vi "Read Sweep Configuration Example.vi"   [LabVIEW 2019, in "SMO.SweepControl.lvclass"]
uses:
  SMO.SweepControl.lvclass
  Typedefs/Enum - Experiments.ctl
  Typedefs/Continuous B Sweep JSON--Cluster.ctl
  Typedefs/Enum - Priority.ctl
  Typedefs/Enum - Action.ctl
  Typedefs/Cluster - ScanControl.ctl
  Typedefs/ScanControl.ctl
  Typedefs/Cluster - ScanParamters.ctl
  Typedefs/ScanParamters.ctl
  Typedefs/Sweep Control JSON--Cluster.ctl
  SMO.Transport/Typedefs/Lockin_Sweep JSON--Cluster.ctl
  SMO.Transport/SMO.Transport.lvclass
  <userlib>/LevyLab/Krohn Hite 7008/typedefs/Input Configuration-Enum.ctl
  <userlib>/LevyLab/Krohn Hite 7008/Instrument.KH7008.lvclass
  <userlib>/LevyLab/Krohn Hite 7008/typedefs/Shunt-Enum.ctl
  <userlib>/LevyLab/Krohn Hite 7008/typedefs/Gain-Enum.ctl
  <userlib>/LevyLab/Krohn Hite 7008/typedefs/Channel-Enum.ctl
  <userlib>/LevyLab/Krohn Hite 7008/typedefs/Coupling-Enum.ctl
  <userlib>/LevyLab/Krohn Hite 7008/typedefs/Filter-Enum.ctl
  <userlib>/LevyLab/Krohn Hite 7008/typedefs/SetAll-Cluster.ctl
  <userlib>/LevyLab/Krohn Hite 7008/typedefs/SetAll-Array.ctl
  <userlib>/LevyLab/Lockin-Multichannel/Instrument.DAQ/Typedefs/REF.Channel--Cluster.ctl
  <userlib>/LevyLab/Lockin-Multichannel/Instrument.DAQ/Instrument.DAQ.lvclass
  <userlib>/LevyLab/Lockin-Multichannel/Instrument.DAQ/Typedefs/REF.Channel--Cluster--Array.ctl
  <userlib>/LevyLab/Lockin-Multichannel/Instrument.DAQ/Typedefs/AO.Channel.Function--Enum.ctl
  <userlib>/LevyLab/Lockin-Multichannel/Instrument.DAQ/Typedefs/AO.Channel--Cluster.ctl
  <userlib>/LevyLab/Lockin-Multichannel/Instrument.DAQ/Typedefs/AO.Channel--Cluster--Array.ctl
  Control Experiment/Typedefs/Wiring Description--v2--cluster.ctl
  Control Experiment/Control Experiment.lvclass
  Control Experiment/Typedefs/Instrument Types--combo.ctl
  Control Experiment/Typedefs/Instrument--enum.ctl
  Control Experiment/Typedefs/Experiment Description--cluster.ctl
panel:
  # "See block diagram for example of how to use ReadSweepConfigurationFile.vi"
types:
  T1 = typedef "SMO.Transport.lvclass/Lockin_Sweep JSON--Cluster.ctl" = cluster{"Sweep Time (s)":dbl, "Sweep Start (V)":dbl, "Sweep End (V)":dbl, "Sweep Channel":i32}
  T2 = typedef "SMO.SweepControl.lvclass/Sweep Control JSON--Cluster.ctl" = cluster{"Experiment":T3, "Repeat Experiment":i32, "Scan control":T4, "Scan parameters":T8}
  T3 = typedef "SMO.SweepControl.lvclass/Enum - Experiments.ctl" = enum16{"IV", "IV_Fast", "THz_DelayLine", "Lockin_Vsg", "Lockin_Sweep", "Lockin_Time", "AI WFM time", "Lockin (experimental)"}
  T4 = typedef "SMO.SweepControl.lvclass/ScanControl.ctl" = T5[]
  T5 = typedef "SMO.SweepControl.lvclass/Cluster - ScanControl.ctl" = cluster{"Priority":T6, "Scan name":T7}
  T6 = typedef "SMO.SweepControl.lvclass/Enum - Priority.ctl" = enum16{"Priority 0", "Priority 1", "Priority 2", "Priority 3", "Priority 4", "Priority 5"}
  T7 = typedef "SMO.SweepControl.lvclass/Enum - Action.ctl" = enum16{"OFF", "time", "Lockin Amplitude", "Lockin Frequency", "Lockin Bias", "Delay", "Strain", "DAQ Bias", "Magnet Field", "Temperature", "MW f1", "MW f2", "MW Amplitude1", "MW Amplitude2"}
  T8 = typedef "SMO.SweepControl.lvclass/ScanParamters.ctl" = T9[]
  T9 = typedef "SMO.SweepControl.lvclass/Cluster - ScanParamters.ctl" = cluster{"Start":dbl, "End":dbl, "Step":dbl, "Rate":dbl, "Waveform type":enum16{"linear", "triangle", "power"}, "wait (ms or K)":dbl, "Address":string, "channel":i32}
  T10 = typedef "SMO.SweepControl.lvclass/Continuous B Sweep JSON--Cluster.ctl" = cluster{"Continuous B Sweep":cluster{"Experiment":T3, "B field values":dbl[]}, "Experiment Description":T11, "Wiring Configuration":T14, "Lockin":cluster{"Channels: AO":T15, "Channels: Lockin":T18}, "Krohn Hite":cluster{"Channel Setting":T20}}
  T11 = typedef "Control Experiment.lvclass/Experiment Description--cluster.ctl" = cluster{"User":string, "Device":string, "Device Path":path, "Device Description":string, "Experiment Path":path, "Experiment Description":string, "Instrument":T12, "Instruments":cluster{"class path":path, "Address":string, "Type":T13}[], "Sweep":cluster{"key":string, "value":variant}[]}
  T12 = typedef "Control Experiment.lvclass/Instrument--enum.ctl" = enum16{"----- AFM/EBL -----", "AGILENT", "CYPHER", "Gemini2", "JEOL", "MFP3D", "----- Cryostat -----", "CF900", "DR200", "MNK", "PPMS (simulated)", "PPMS 1", "PPMS 2", "PPMS 3", "----- Optics -----", "THz 1 (Element 2/Montana)", "THz 2 (Tsunami/Janis)"}
  T13 = typedef "Control Experiment.lvclass/Instrument Types--combo.ctl" = string
  T14 = typedef "Control Experiment.lvclass/Wiring Description--v2--cluster.ctl" = cluster{"AI":cluster{"Channel":u32, "Gain":dbl}, "Device":cluster{"Electrode":string, "Label":string, "Type":string}, "KH":cluster{"Channel":string, "Configuration":string, "Gain":u32, "Shunt Resistor":u32}, "AO":cluster{"Channel":u32, "Gain":dbl}}
  T15 = typedef "Instrument.DAQ.lvclass/AO.Channel--Cluster--Array.ctl" = T16[]
  T16 = typedef "Instrument.DAQ.lvclass/AO.Channel--Cluster.ctl" = cluster{"Enable?":bool, "Channel":i32, "Amplitude":dbl, "Offset":dbl, "Frequency":dbl, "Phase":dbl, "Function":T17, "Sweeping?":bool}
  T17 = typedef "Instrument.DAQ.lvclass/AO.Channel.Function--Enum.ctl" = enum16{"Sine", "Triangle", "Square"}
  T18 = typedef "Instrument.DAQ.lvclass/REF.Channel--Cluster--Array.ctl" = T19[]
  T19 = typedef "Instrument.DAQ.lvclass/REF.Channel--Cluster.ctl" = cluster{"Enable?":bool, "Channel":i32, "Frequency":dbl, "Phase":dbl, "TC":dbl, "Roll-Off":i32}
  T20 = typedef "Instrument.KH7008.lvclass/SetAll-Array.ctl" = T21[]
  T21 = typedef "Instrument.KH7008.lvclass/SetAll-Cluster.ctl" = cluster{"Channel":T22, "Gain":T23, "Bandwidth Filter":T24, "Shunt Resistor":T25, "Coupling":T26, "Input Config":T27}
  T22 = typedef "Instrument.KH7008.lvclass/Channel-Enum.ctl" = enum16{"Channel 1", "Channel 2", "Channel 3", "Channel 4", "Channel 5", "Channel 6", "Channel 7", "Channel 8"}
  T23 = typedef "Instrument.KH7008.lvclass/Gain-Enum.ctl" = enum16{"1x", "10x", "100x", "1000x"}
  T24 = typedef "Instrument.KH7008.lvclass/Filter-Enum.ctl" = enum16{"OFF", "ON"}
  T25 = typedef "Instrument.KH7008.lvclass/Shunt-Enum.ctl" = enum16{"Open", "50 Ohms", "500 Ohms", "5k Ohms", "50k Ohms", "10M Ohm"}
  T26 = typedef "Instrument.KH7008.lvclass/Coupling-Enum.ctl" = enum16{"AC", "DC"}
  T27 = typedef "Instrument.KH7008.lvclass/Input Configuration-Enum.ctl" = enum16{"Ground", "SE+ (-gnd)", "SE- (+gnd)", "Differential"}
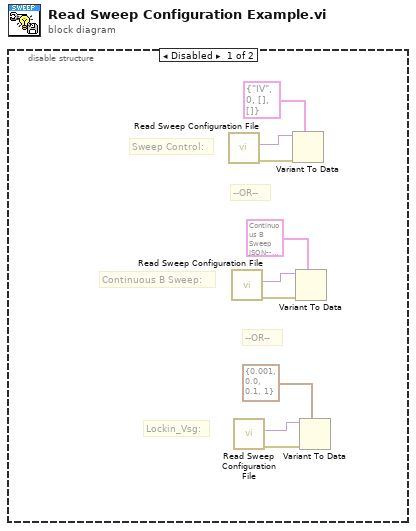
[diagram p0: block diagram]
diagram:
  n1 = disable-structure shown="Disabled" {
    frame Disabled {
      # "Lockin_Vsg:"
      # "Continuous B Sweep:"
      # "Sweep Control:"
      # "--OR--"
      # "--OR--"
      n2 = call "Read Sweep Configuration File.vi"() -> ("error out"=w9:errorcluster, "Data"=w5:variant)  [unwired: 9 in, 1 out]
      n3 = call "Read Sweep Configuration File.vi"() -> ("error out"=w6:errorcluster, "Data"=w4:variant)  [unwired: 9 in, 1 out]
      n4 = call "Read Sweep Configuration File.vi"() -> ("error out"=w8:errorcluster, "Data"=w7:variant)  [unwired: 9 in, 1 out]
      n5 = Variant To Data(error in=w9, type=T2 {"Experiment"=enum."IV", "Repeat Experiment"=0, "Scan control"=[], "Scan parameters"=[]} ("SweepControl"), Variant=w5) -> ()  [unwired: 2 out]
      n6 = Variant To Data(error in=w6, type=T10 {"Continuous B Sweep"={"Experiment"=enum."IV", "B field values"=[]}, "Experiment Description"={"User"="", "Device"="", "Device Path"=path "", "Device Description"="", "Experiment Path"=path "", "Experiment Description"="", "Instrument"=enum."----- AFM/EBL -----", "Instruments"=[], "Sweep"=[]}, "Wiring Configuration"={"AI"={"Channel"=0, "Gain"=0.0}, "Device"={"Electrode"="", "Label"="", "Type"=""}, "KH"={"Channel"="", "Configuration"="", "Gain"=0, "Shunt Resistor"=0}, "AO"={"Channel"=0, "Gain"=0.0}}, "Lockin"={"Channels: AO"=[], "Channels: Lockin"=[]}, "Krohn Hite"={"Channel Setting"=[]}} ("ContinuousBSweep"), Variant=w4) -> ()  [unwired: 2 out]
      n7 = Variant To Data(error in=w8, type=T1 {"Sweep Time (s)"=0.001, "Sweep Start (V)"=0.0, "Sweep End (V)"=0.1, "Sweep Channel"=1} ("LockinVsg Sweep"), Variant=w7) -> ()  [unwired: 2 out]
    }
    frame Enabled {
    }
  }
